vi "Global target position.vi"() -> ()   [LabVIEW 2012, in "StageSPIM.lvclass"]
uses:
  StageSPIM/StageSPIM.lvclass
panel:
  in  "global target position":dbl[](array[numeric])
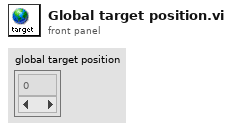
[diagram p1: front panel]
diagram:
